vi "Car Wash Empty Array (SubVI).vi"(8 "error in (no error)":errorcluster, 10 "Array in":string[](array[string]), 11 "Array reference in":refnum<vi>) -> (0 "error out":errorcluster, 2 "Array out":string[](array[string]), 3 "Array reference out":refnum<vi>)   [LabVIEW 2018]
panel:
  # "Input Values"
  # "Output Values"
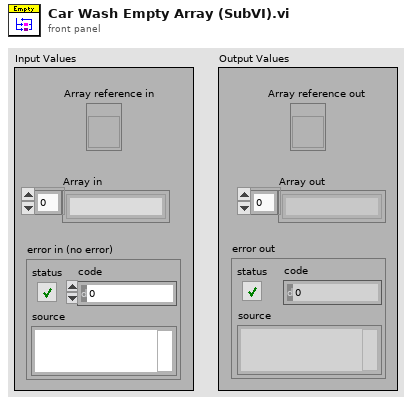
[diagram p1: front panel]
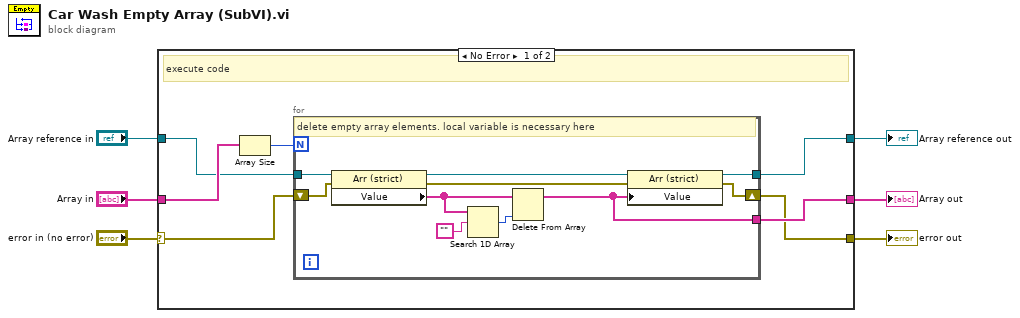
[diagram p0: block diagram]
diagram:
  n1 = case shown="No Error" "error in (no error)" {
    selector: "error in (no error)" -> [w9 w26]
    tunnel: "Array in" -> [w13 w25]
    tunnel: "Array reference in" -> [w11 w24]
    tunnel: [w8 w26] -> w3
    tunnel: [w10 w25] -> w2
    tunnel: [w7 w24] -> w1
    frame No Error {
      # "execute code"
      n2 = Array Size(array=w13) -> (size(s)=w12:i32)
      n3 = for {
        N: w12 -> [_]
        tunnel: w11 -> [w20]
        tunnel: [w18] -> w10
        shift-right: [w15] -> w8
        shift-left: w9 -> [w17]
        tunnel: [w14] -> w7
        # "delete empty array elements. local variable is necessary here"
        n4 = property class="Arr (strict)"(reference=w20, error in=w17) -> (reference out=w19:refnum<vi>, error out=w16:errorcluster, "Value"=w22:string[])
        n5 = Search 1D Array(1D array=w22, element="") -> (index of element=w21:i32)  [unwired: 1 in]
        n6 = Delete From Array "Delete From Array"(array=w22, index=w21) -> (array with subset deleted=w18:string[])  [unwired: 1 in, 1 out]
        n7 = property class="Arr (strict)"(reference=w19, error in=w16, "Value"=w18) -> (reference out=w14:refnum<vi>, error out=w15:errorcluster)
      }
    }
    frame Error {
      # "do nothing"
    }
  }
  "error out" <- w3
  "Array out" <- w2
  "Array reference out" <- w1
